vi "WaitStop.vi"(8 "error in (no error)":errorcluster, 11 "VISA resource name":refnum<visa-resource-name>) -> (0 "error out":errorcluster, 2 "Moving":bool)   [LabVIEW 2012, in "Micos_uic.lvlib"]
doc: "Performs an instrument error query before terminating the software connection to the instrument."
uses:
  Micos_uic.lvlib
  Position_Micos.vi
panel:
  out "still?":bool
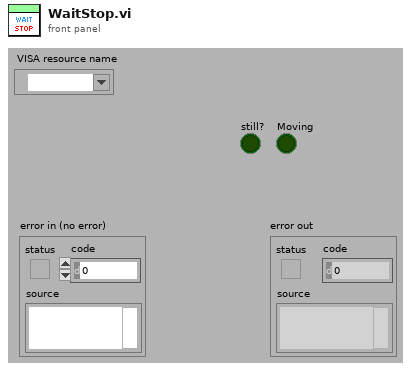
[diagram p1: front panel]
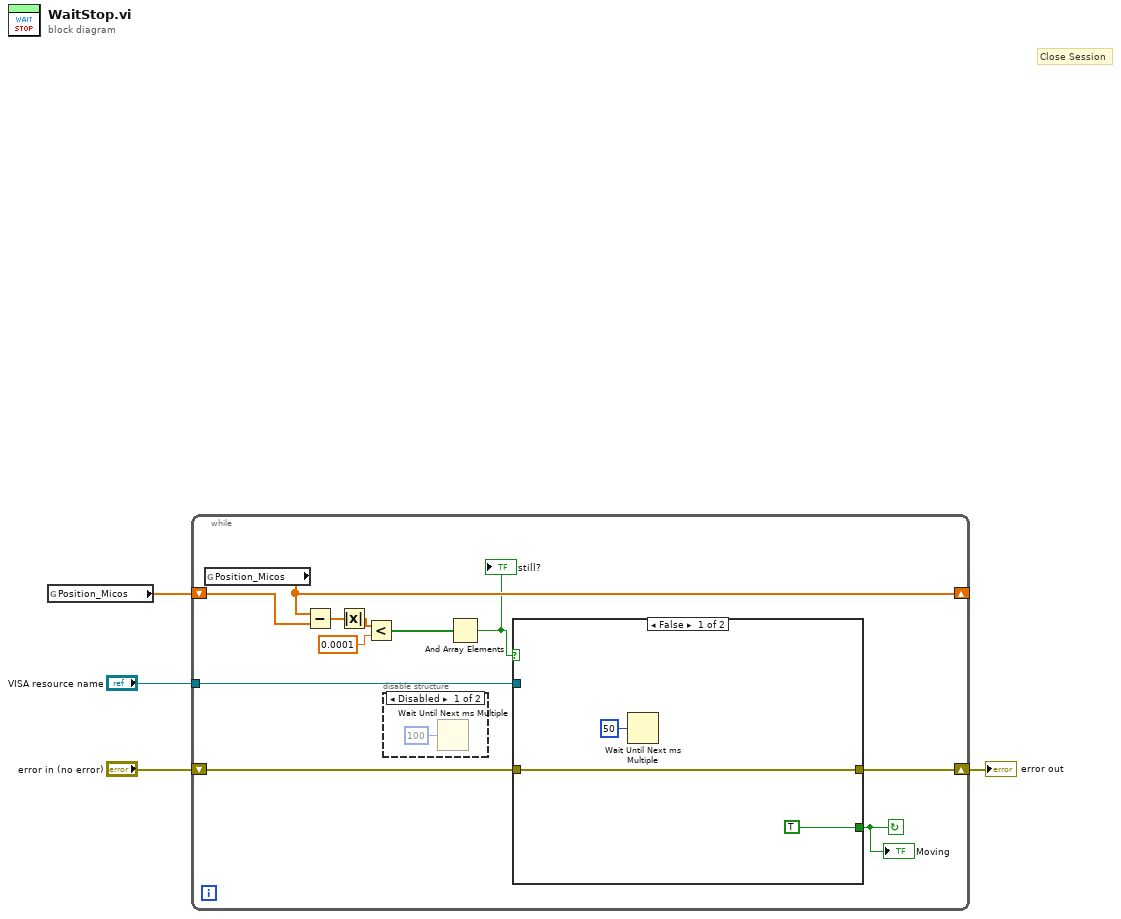
[diagram p0: block diagram]
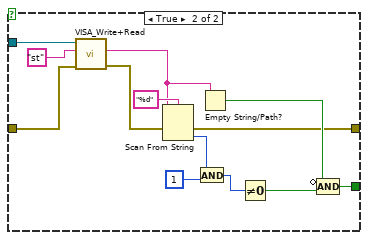
[diagram p3: hidden frame]
diagram:
  # "Close Session"
  n1 = global read "Position_Micos.vi" "Position_Micos"() -> (w1:dbl[])
  n2 = while {
    tunnel: "VISA resource name" -> [w15]
    shift-right: [w14] -> w3
    shift-left: "error in (no error)" -> [w13]
    shift-right: [w12] -> _
    shift-left: w1 -> [w11]
    stop <- w5 continue-if-true
    n3 = global read "Position_Micos.vi" "Position_Micos"() -> (w12:dbl[])
    n4 = Subtract(x=w12, y=w11) -> (x-y=w9:dbl[])
    n5 = Absolute Value(x=w9) -> (abs(x)=w6:dbl[])
    n6 = Less?(x=w6, y=0.0001) -> (x < y?=w7:bool[])
    n7 = disable-structure shown="Disabled" {
      frame Disabled {
        n8 = Wait Until Next ms Multiple(millisecond multiple=u32 100) -> ()  [unwired: 1 out]
      }
      frame Enabled {
      }
    }
    n9 = And Array Elements(Boolean array=w7) -> (logical AND=w10:bool)
    "still?" <- w10
    n10 = case shown="False" w10 {
      tunnel: w15 -> [_ w31]
      tunnel: [w19 w30] -> w14
      tunnel: w13 -> [w19 w29]
      tunnel: [TRUE w28] -> w5
      frame False {
        n11 = Wait Until Next ms Multiple(millisecond multiple=u32 50) -> ()  [unwired: 1 out]
      }
      frame True {
        n12 = call "VISA_Write+Read.vi"("error in (no error)"=w29, "Write Buffer"="st" ("string"), "VISA resource name"=w31) -> ("error out"=w25:errorcluster, "readout"=w20:string)  [unwired: 6 in, 1 out]
        n13 = Scan From String(format string="%d", input string=w20, error in=w25) -> (error out=w30:errorcluster, output 1=w24:i32)  [unwired: 2 in, 2 out]
        n14 = And(x=w24, y=1) -> (x .and. y?=w22:i32)
        n15 = Empty String/Path?(string/path=w20) -> (empty?=w32:bool)
        n16 = Not Equal To 0?(x=w22) -> (x != 0?=w21:bool)
        n17 = Compound Arithmetic op=AND(invert w32, w21) -> (w28:bool)
      }
    }
    "Moving" <- w5
  }
  "error out" <- w3
